vi "SaveBattleIntoDB.vi"(8 "error in (no error)":errorcluster, 11 "ClashRoyale in":refnum<class "StashRoyale.lvclass">) -> (0 "error out":errorcluster, 3 "ClashRoyale out":refnum<class "StashRoyale.lvclass">)   [LabVIEW 2020, in "StashRoyale.lvclass"]
uses:
  StashRoyale.lvclass
  StashRoyale.lvclass/StashRoyale.ctl
  <vilib>/drjdpowell/SQLite Library/SQL Connection/Execute SQL (No results).vi
  <vilib>/drjdpowell/SQLite Library/SQLite.lvlib
  <vilib>/drjdpowell/SQLite Library/SQL Connection/Connection.lvclass
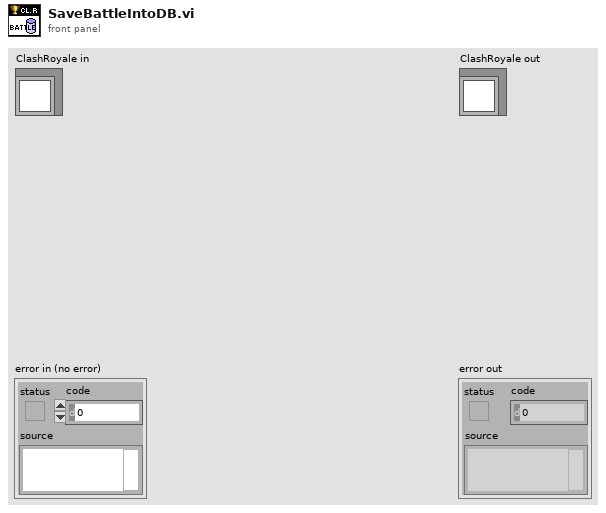
[diagram p1: front panel]
types:
  T1 = typedef "StashRoyale.lvclass/ctl_BattleLog.ctl" = cluster{"type":string, "battleTime":string, "isLadderTournament":bool, "arena":cluster{"id":u32, "name":string}, "gameMode":cluster{"id":u32, "name":string}, "deckSelection":string, "team":T2[]}
  T2 = typedef "ctl_Team.ctl" = cluster{"tag":string, "name":string, "startingTrophies":u16, "trophyChange":i16, "kingTowerHitPoints":u16, "crowns":u16, "elixirLeaked":sgl, "cards":T3[]}
  T3 = typedef "StashRoyale.lvclass/ctl_CardTeam.ctl" = cluster{"id":u32, "level":u8}
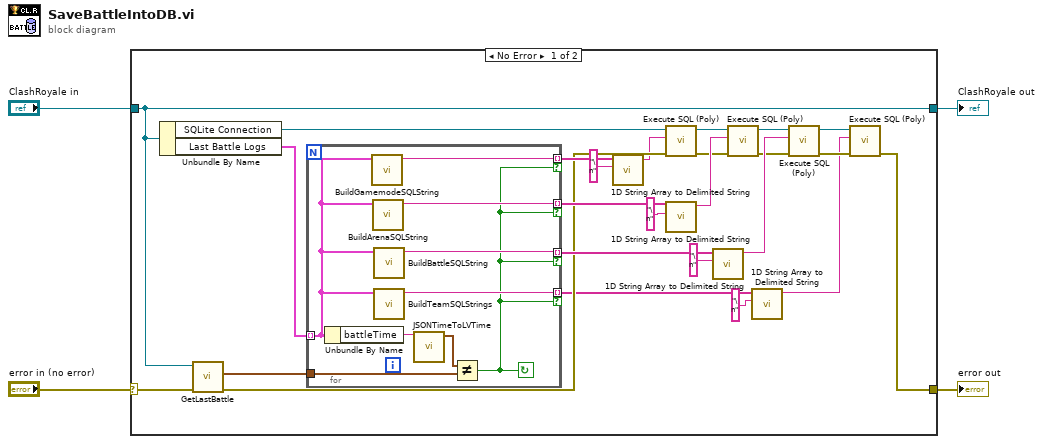
[diagram p0: block diagram]
diagram:
  n1 = case shown="No Error" "error in (no error)" {
    selector: "error in (no error)" -> [w27 w40]
    tunnel: [w5 w40] -> w3
    tunnel: [w26 w39] -> w1
    tunnel: "ClashRoyale in" -> [w26 w39]
    frame No Error {
      n2 = Unbundle By Name(w26) -> ("SQLite Connection"=w18:refnum<class "Connection.lvclass">, "Last Battle Logs"=w24:T1[])
      n3 = call "GetLastBattle.vi"("error in (no error)"=w27, "ClashRoyale in"=w26) -> ("error out"=w17:errorcluster, "Last Battle Time"=w25:timestamp)  [unwired: 7 in, 1 out]
      n4 = for {
        tunnel: w24 -> [w32] mode=indexing
        tunnel: w25 -> [w36]
        tunnel: [w35] -> w23 mode=indexing if=w30
        tunnel: [w34] -> w19 mode=indexing if=w30
        tunnel: [w33] -> w20 mode=indexing if=w30
        tunnel: [w31] -> w9 mode=indexing if=w30
        stop <- w30 continue-if-true
        n5 = Unbundle By Name(w32) -> ("battleTime"=w38:string)
        n6 = call "BuildGamemodeSQLString.vi"("BattleLog"=w32) -> ("SQL INSERT request"=w34:string)  [unwired: 10 in]
        n7 = call "BuildArenaSQLString.vi"("BattleLog"=w32) -> ("SQL INSERT request"=w33:string)  [unwired: 10 in]
        n8 = call "BuildBattleSQLString.vi"("BattleLog"=w32) -> ("SQL INSERT request"=w35:string)  [unwired: 10 in]
        n9 = call "BuildTeamSQLStrings.vi"("BattleLog"=w32) -> ("Team SQL INSERT request"=w31:string)  [unwired: 10 in]
        n10 = call "JSONTimeToLVTime.vi"("JSON time stamp"=w38) -> ("LV time stamp"=w37:timestamp)  [unwired: 10 in]
        n11 = Not Equal?(x=w37, y=w36) -> (x != y?=w30:bool)
      }
      n12 = call <vilib>:"1D String Array to Delimited String.vi"("delimiter"="\n", "string array"=w19) -> ("delimited string"=w16:string)  [unwired: 9 in]
      n13 = call-poly <vilib>:"Execute SQL (Poly).vi"("error in (no error)"=w17, "SQL"=w16, "SQLite Connection in"=w18) -> ("error out"=w13:errorcluster, "SQLite Connection"=w14:refnum<class "Connection.lvclass">)  [unwired: 7 in]
      n14 = call <vilib>:"1D String Array to Delimited String.vi"("delimiter"="\n", "string array"=w20) -> ("delimited string"=w15:string)  [unwired: 9 in]
      n15 = call <vilib>:"1D String Array to Delimited String.vi"("delimiter"="\n", "string array"=w23) -> ("delimited string"=w29:string)  [unwired: 9 in]
      n16 = call-poly <vilib>:"Execute SQL (Poly).vi"("error in (no error)"=w13, "SQL"=w15, "SQLite Connection in"=w14) -> ("error out"=w12:errorcluster, "SQLite Connection"=w11:refnum<class "Connection.lvclass">)  [unwired: 7 in]
      n17 = call <vilib>:"1D String Array to Delimited String.vi"("delimiter"="\n", "string array"=w9) -> ("delimited string"=w6:string)  [unwired: 9 in]
      n18 = call-poly <vilib>:"Execute SQL (Poly).vi"("error in (no error)"=w12, "SQL"=w29, "SQLite Connection in"=w11) -> ("error out"=w8:errorcluster, "SQLite Connection"=w7:refnum<class "Connection.lvclass">)  [unwired: 7 in]
      n19 = call-poly <vilib>:"Execute SQL (Poly).vi"("error in (no error)"=w8, "SQL"=w6, "SQLite Connection in"=w7) -> ("error out"=w5:errorcluster)  [unwired: 7 in, 1 out]
    }
    frame Error {
    }
  }
  "error out" <- w3
  "ClashRoyale out" <- w1
